vi "Find Test Cases in LVProj.vi"(8 "error in (no error)":errorcluster, 11 "Project Path":path) -> (0 "error out":errorcluster, 2 "Test Class paths":path[](array[path]))   [LabVIEW 2020, in "LUnit Test Suite V2.lvclass"]
uses:
  LUnit Test Suite V2.lvclass
  LUnit Test Case/LUnit Test Case V2.lvclass
  LUnit Test Suite V2.lvclass/LUnit Test Suite V2.ctl
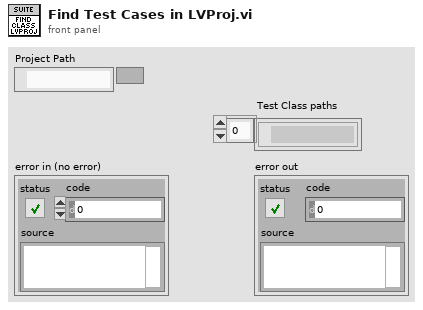
[diagram p1: front panel]
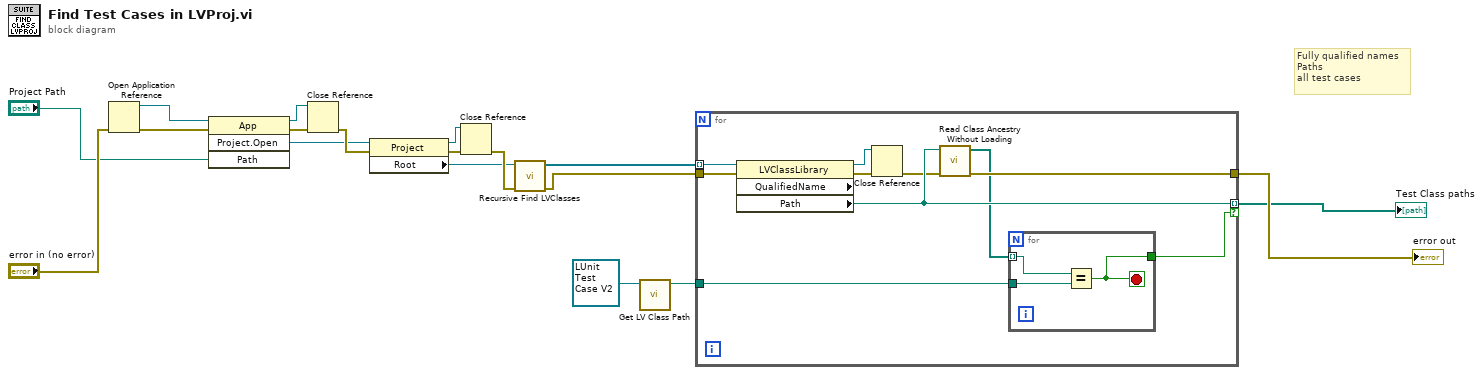
[diagram p0: block diagram]
diagram:
  # "Fully qualified names\nPaths\nall test cases"
  n1 = Open Application Reference(8:"error in (no error)") -> (0:w8:errorcluster, 3:w7:refnum<vi>)  [unwired: 3 in]
  n2 = invoke class="App" method="Project.Open"(reference=w7, error in=w8, "Path"="Project Path") -> (reference out=w10:refnum<vi>, error out=w9:errorcluster, "Project:Open"=w11:refnum<vi>)  [unwired: 1 in, 1 out]
  n3 = Close Reference(reference=w10, error in (no error)=w9) -> (error out=w12:errorcluster)
  n4 = property class="Project"(reference=w11, error in=w12) -> (reference out=w18:refnum<vi>, error out=w13:errorcluster, "Root"=w3:refnum<vi>)
  n5 = Close Reference(reference=w18, error in (no error)=w13) -> (error out=w17:errorcluster)
  n6 = call "Recursive Find LVClasses.vi"("error in (no error)"=w17, "reference"=w3) -> ("error out"=w4:errorcluster, "Class References"=w14:refnum<vi>[])  [unwired: 8 in]
  n7 = call <vilib>:"Get LV Class Path.vi"("object"=refnum<class "LUnit Test Case V2.lvclass"> refnum ("LUnit Test Case V2.lvclass")) -> ("class path"=w1:path)  [unwired: 9 in, 1 out]
  n8 = for {
    tunnel: w14 -> [w28] mode=indexing
    tunnel: w4 -> [w27]
    tunnel: [w20] -> w16
    tunnel: [w24] -> w5 mode=indexing if=w22
    tunnel: w1 -> [w23]
    n9 = property class="LVClassLibrary" props=["QualifiedName", "Path"](reference=w28, error in=w27) -> (reference out=w25:refnum<vi>, error out=w26:errorcluster, "Path"=w24:path)  [unwired: 1 out]
    n10 = Close Reference(reference=w25, error in (no error)=w26) -> (error out=w21:errorcluster)
    n11 = call <vilib>:"Read Class Ancestry Without Loading.vi"("error in (no error)"=w21, "LabVIEW Class Path"=w24) -> ("error out"=w20:errorcluster, "Class Ancestry"=w19:path[])  [unwired: 8 in]
    n12 = for {
      tunnel: w19 -> [w30] mode=indexing
      tunnel: w23 -> [w31]
      tunnel: [w29] -> w22
      stop <- w29 stop-if-true
      n13 = Equal?(x=w30, y=w31) -> (x = y?=w29:bool)
    }
  }
  "error out" <- w16
  "Test Class paths" <- w5
